vi "set_wavelength_python.vi"(8 "error in (no error)":errorcluster, 10 "wavelength":dbl, 11 "Addr":string) -> (0 "error out":errorcluster, 3 "Addr out":string)   [LabVIEW 2018]
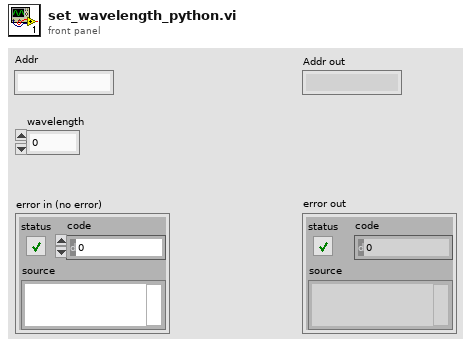
[diagram p1: front panel]
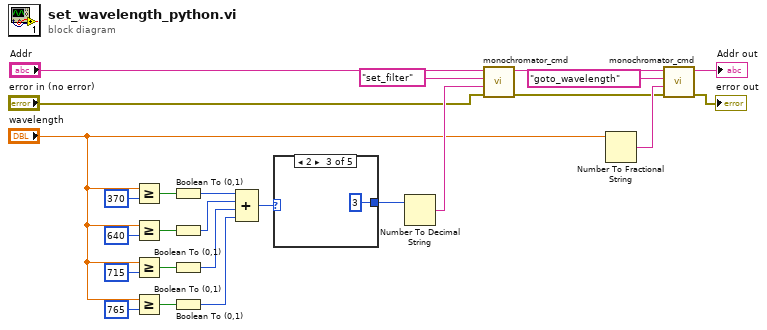
[diagram p0: block diagram]
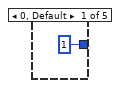
[diagram p2: hidden frame]
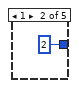
[diagram p3: hidden frame]
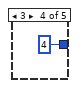
[diagram p4: hidden frame]
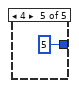
[diagram p5: hidden frame]
diagram:
  n1 = Greater Or Equal?(x="wavelength", y=370) -> (x >= y?=w21:bool)
  n2 = Greater Or Equal?(x="wavelength", y=640) -> (x >= y?=w20:bool)
  n3 = Greater Or Equal?(x="wavelength", y=715) -> (x >= y?=w19:bool)
  n4 = Greater Or Equal?(x="wavelength", y=765) -> (x >= y?=w18:bool)
  n5 = Boolean To (0,1)(Boolean=w21) -> (0, 1=w17:i16)
  n6 = Boolean To (0,1)(Boolean=w20) -> (0, 1=w16:i16)
  n7 = Boolean To (0,1)(Boolean=w19) -> (0, 1=w15:i16)
  n8 = Boolean To (0,1)(Boolean=w18) -> (0, 1=w14:i16)
  n9 = Compound Arithmetic op=ADD(w17, w16, w15, w14) -> (w13:i16)
  n10 = case shown="2" w13 {
    tunnel: [1 2 3 4 5] -> w11
    frame 0, Default {
    }
    frame 1 {
    }
    frame 2 {
    }
    frame 3 {
    }
    frame 4 {
    }
  }
  n11 = Number To Decimal String(number=w11) -> (decimal integer string=w10:string)  [unwired: 1 in]
  n12 = call "monochromator_cmd.vi"("error in (no error)"="error in (no error)", "Parameter"=w10, "Command"="set_filter", "Addr in"="Addr") -> ("error out"=w3:errorcluster, "Addr out"=w6:string)  [unwired: 4 in, 2 out]
  n13 = Number To Fractional String(number="wavelength") -> (F-format string=w4:string)  [unwired: 3 in]
  n14 = call "monochromator_cmd.vi"("error in (no error)"=w3, "Parameter"=w4, "Command"="goto_wavelength", "Addr in"=w6) -> ("error out"=→"error out":errorcluster, "Addr out"=→"Addr out":string)  [unwired: 4 in, 2 out]
